vi "corrected_turn_rate.vi"(9 "Time between reading":dbl=0.125, 10 "Previous Heading":dbl, 11 "Current Heading":dbl) -> (1 "difference":dbl, 2 "Previous Heading":dbl, 3 "Turn rate":dbl)   [LabVIEW 2009]
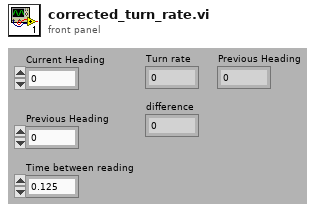
[diagram p1: front panel]
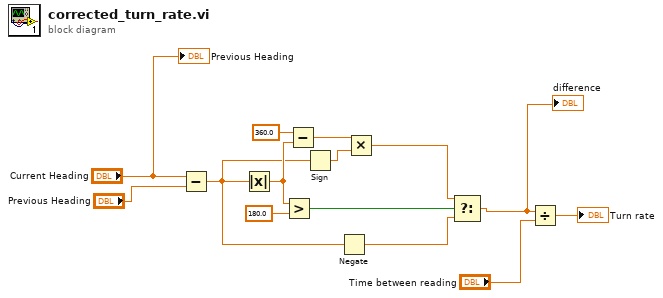
[diagram p0: block diagram]
diagram:
  n1 = Subtract(x="Current Heading", y="Previous Heading") -> (x-y=w2:dbl)
  n2 = Absolute Value(x=w2) -> (abs(x)=w4:dbl)
  n3 = Greater?(x=w4, y=180.0) -> (0:w9:bool)
  n4 = Subtract(x=360.0, y=w4) -> (x-y=w7:dbl)
  n5 = Sign(1:w2) -> (0:w6:dbl)
  n6 = Negate(x=w2) -> (-x=w3:dbl)
  n7 = Multiply(x=w7, y=w6) -> (x*y=w5:dbl)
  n8 = Select(t=w5, s=w9, f=w3) -> (s? t:f=w1:dbl)
  "difference" <- w1
  n9 = Divide(x=w1, y="Time between reading") -> (x/y=→"Turn rate":dbl)
  "Previous Heading" <- "Current Heading"
